vi "convert lines to channels.vi"(8 "error in (no error)":errorcluster, 11 "Lines in":T1[](array[typedef])) -> (0 "error out":errorcluster, 3 "channels out":refnum<class "TBM channel.lvclass">[](array[class]))   [LabVIEW 2013, in "Shared Memory configuration.lvclass"]
uses:
  Shared Memory configuration.lvclass
  Line.ctl
  <vilib>/NI/Tag Bus Module Framework/channel/TBM channel.lvclass
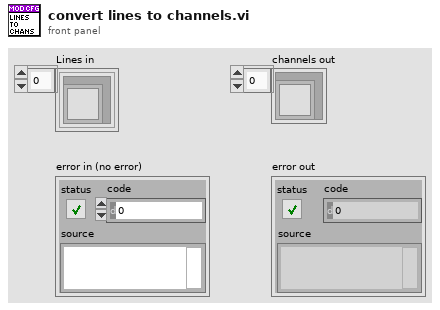
[diagram p1: front panel]
types:
  T1 = typedef "Shared Memory configuration.lvclass/Line.ctl" = cluster{"channel":refnum<class "TBM channel.lvclass">}
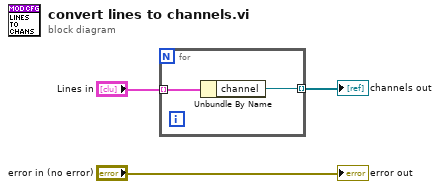
[diagram p0: block diagram]
diagram:
  n1 = for {
    tunnel: "Lines in" -> [w5] mode=indexing
    tunnel: [w4] -> w2 mode=indexing
    n2 = Unbundle By Name(w5) -> ("channel"=w4:refnum<class "TBM channel.lvclass">)
  }
  "channels out" <- w2
  "error out" <- "error in (no error)"
